vi "电机数据.vi"() -> ()   [LabVIEW 2017]
uses:
  LVMQTT/Controls/Connect_Flags.ctl
  LVMQTT/Controls/QoS.ctl
  <vilib>/Platform/TimedLoop/XDataNode/timing_clust.ctl
  <vilib>/Platform/TimedLoop/XDataNode/nitl_modes.ctl
  <vilib>/Platform/TimedLoop/XDataNode/wakeup.ctl
  <vilib>/Platform/TimedLoop/XDataNode/XDataNode.xnode
  LVMQTT/MQTT_Functions.lvlib
  <vilib>/Platform/TimedLoop/XDataNode/XDNodeRunTimeDep.lvlib
panel:
  out "波形":cluster{"扭矩":dbl, "扭矩":dbl, "扭矩":dbl}(graph)
  out "功率":dbl format="%#_10f"
  out "速度":dbl format="%#_10f"
  out "扭矩":dbl format="%#_10f"
  out "字符串":string
  in  "MQTT Broker":cluster{"address (IP)":string, "port":u16}={"address (IP)"="169.254.84.131", "port"=1883}
  out "period":u32
  out "period 2":u32
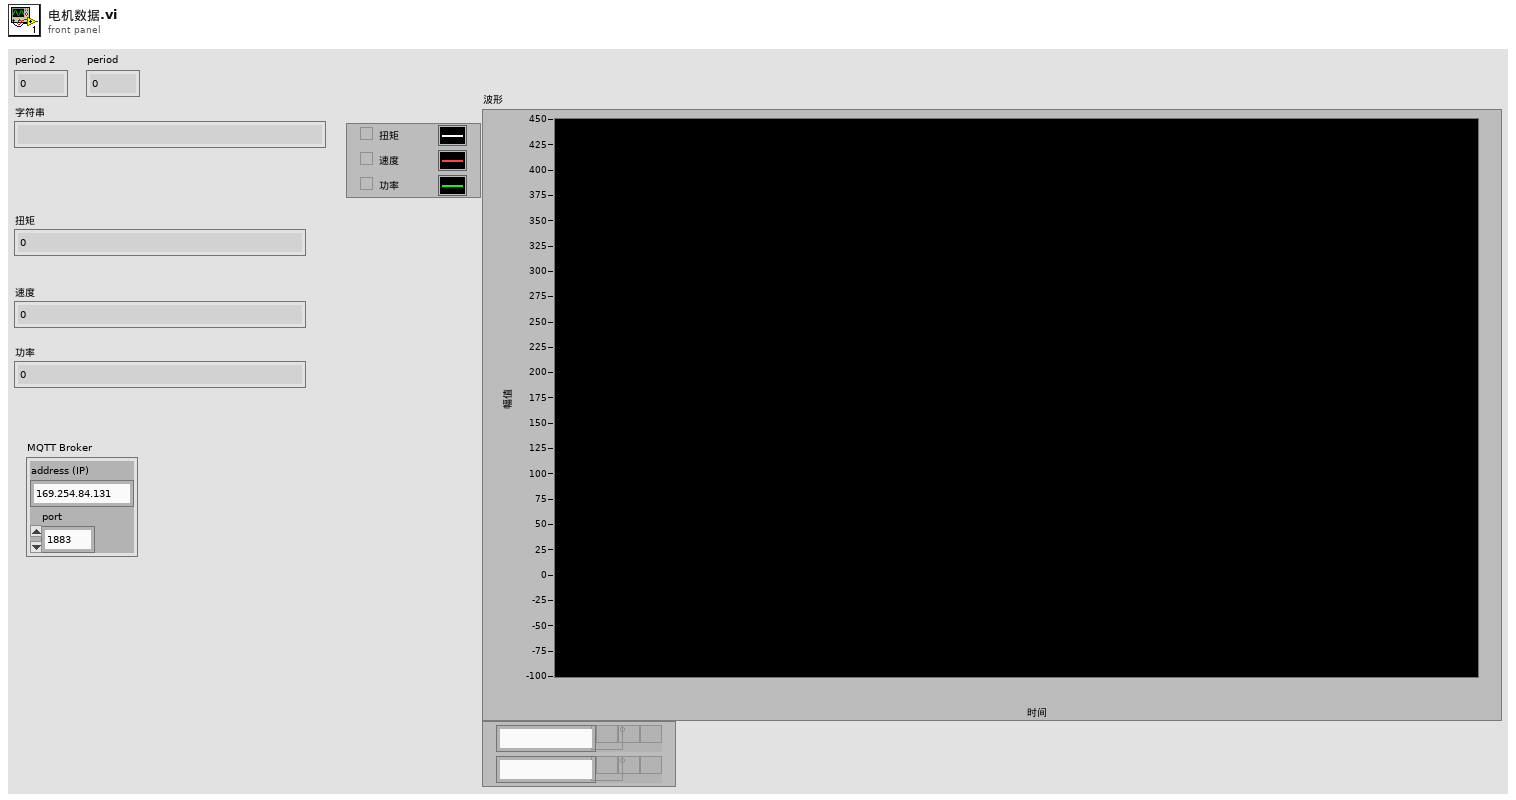
[diagram p1: front panel]
types:
  T1 = typedef "MQTT_Functions.lvlib/QoS.ctl" = enum8{"At most once", "At least once", "Exactly once", "Reserved"}
  T2 = typedef "MQTT_Functions.lvlib/Connect_Flags.ctl" = cluster{"user name":bool, "password":bool, "will retain":bool, "will flag":bool, "clean session":bool, "reserved":bool, "will QoS":T1}
  T3 = typedef "XDNodeRunTimeDep.lvlib/timing_clust.ctl" = cluster{"Expected End [f-1]":u64, "Actual End [f-1]":u64, "Finished Late? [f-1]":bool, "Expected End [i-1]":u64, "Actual End [i-1]":u64, "Finished Late? [i-1]":bool, "Expected Start [i]":u64, "Actual Start [i]":u64, "Expected Start [f]":u64, "Actual Start [f]":u64, "Source Name":string, "Structure Name":string, "Period":i64, "Deadline":i64, "Offset":i64, "Start":i64, "Priority":i32, "Timeout":i32, "Mode":T4, "Wakeup Reason":T5, "Error":errorcluster, "Source Type":string, "Secondary Source Type":string, "Global End Time":u64, "Global Start Time":u64, "Frame Duration":u64, "Iteration Duration":u64, "Assigned CPU":i32, "I/O Scan Engine Mode":u32}
  T4 = typedef "XDNodeRunTimeDep.lvlib/nitl_modes.ctl" = enum32{"No Change", "Process missed periods, maintain original phase", "Discard missed periods, maintain original phase", "Process missed periods, ignore original phase", "Discard missed periods, ignore original phase"}
  T5 = typedef "XDNodeRunTimeDep.lvlib/wakeup.ctl" = enum32{"Normal", "Aborted", "Asynchronous wakeup", "Timing source error", "Timed loop error", "Timeout"}
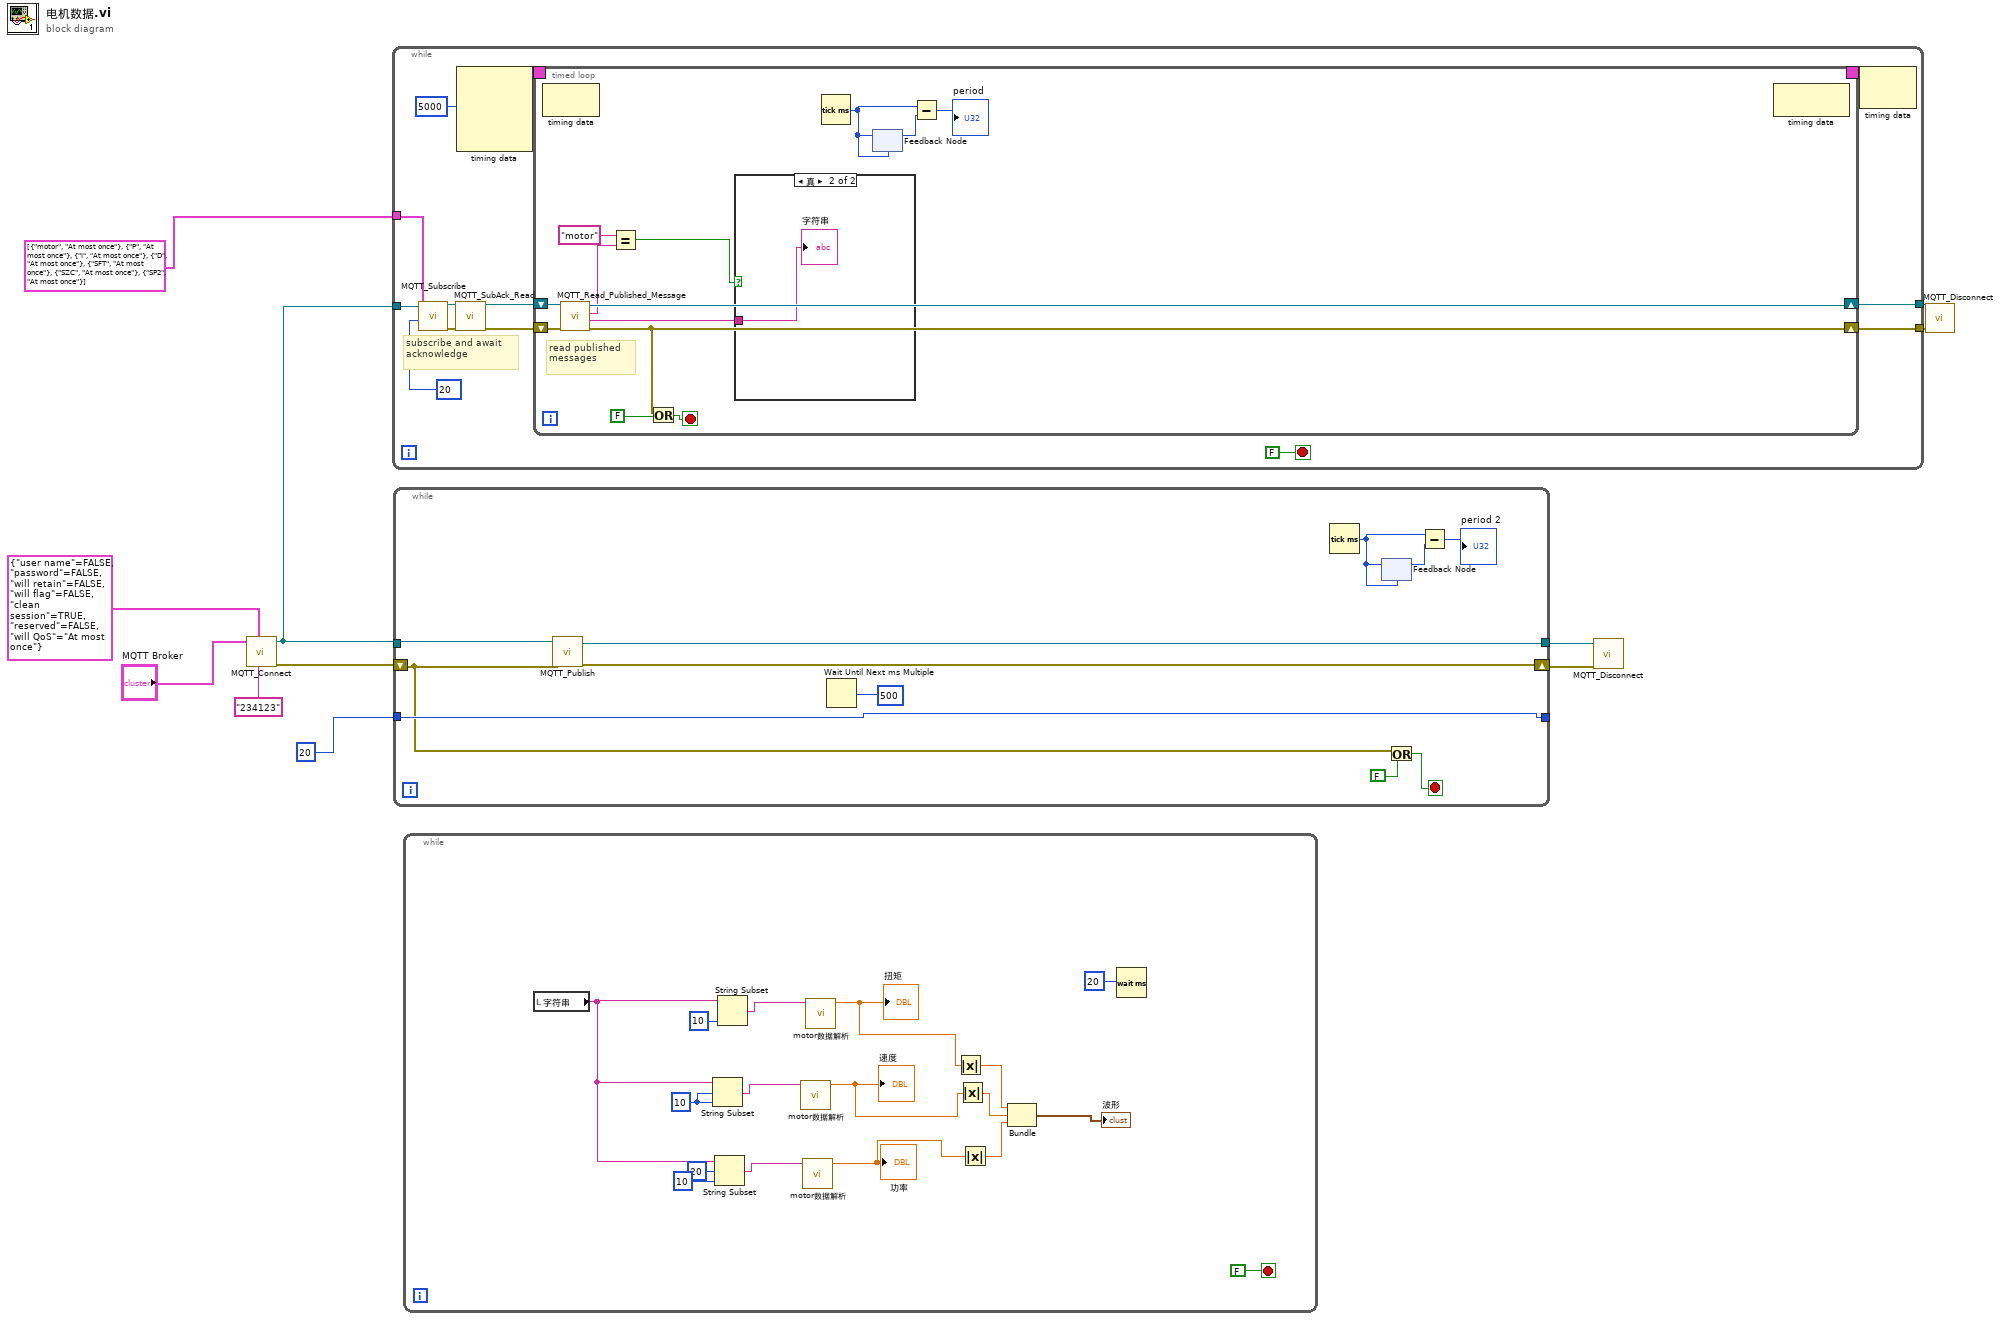
[diagram p0: block diagram]
diagram:
  n1 = call "MQTT_Connect.vi"("Client ID"="234123", "Connect Flags"=T2 {"user name"=FALSE, "password"=FALSE, "will retain"=FALSE, "will flag"=FALSE, "clean session"=TRUE, "reserved"=FALSE, "will QoS"=enum."At most once"}, "MQTT Broker"="MQTT Broker") -> ("error out"=w7:errorcluster, "connection ID out"=w6:refnum<k5>)  [unwired: 6 in, 1 out]
  n2 = while {
    tunnel: w6 -> [w19]
    tunnel: [w18] -> w3
    tunnel: [w17] -> w2
    tunnel: cluster{"Topic":string, "QoS":T1}[] [{"Topic"="motor", "QoS"=enum."At most once"}, {"Topic"="P", "QoS"=enum."At most once"}, {"Topic"="I", "QoS"=enum."At most once"}, {"Topic"="D", "QoS"=enum."At most once"}, {"Topic"="SFT", "QoS"=enum."At most once"}, {"Topic"="SZC", "QoS"=enum."At most once"}, {"Topic"="SP2", "QoS"=enum."At most once"}] ("Subscription Info Array") -> [w16]
    stop <- FALSE stop-if-true
    # "subscribe and await\nacknowledge"
    n3 = call "MQTT_Subscribe.vi"("Message ID"=u16 20, "Subscription Info Array"=w16, "connection ID"=w19) -> ("error out"=w22:errorcluster, "connection ID out"=w23:refnum<k5>)  [unwired: 7 in]
    n4 = call "MQTT_SubAck_Read.vi"("error in (no error)"=w22, "connection ID"=w23) -> ("error out"=w21:errorcluster, "connection ID out"=w20:refnum<k5>)  [unwired: 7 in, 1 out]
    n5 = node-c288(i64 5000 ("周期")) -> (w14:T3)  [unwired: 3 in]
    n6 = timed-loop {
      shift-right: [w29] -> w17
      shift-left: w21 -> [w37]
      shift-right: [w30] -> w18
      shift-left: w20 -> [w36]
      timing: w14 -> [_]
      timing-out: [_] -> w13
      stop <- w35 stop-if-true
      # "read published\nmessages"
      n7 = node-c288() -> ()  [unwired: 1 in, 1 out]
      n8 = call "MQTT_Read_Published_Message.vi"("error in (no error)"=w37, "connection ID"=w36) -> ("error out"=w29:errorcluster, "Message"=w28:string, "Topic Name"=w27:string, "connection ID out"=w30:refnum<k5>)  [unwired: 4 in, 2 out]
      n9 = Equal?(x="motor", y=w27) -> (x = y?=w25:bool)
      n10 = Or(x=w29, y=FALSE) -> (x .or. y?=w35:bool)
      n11 = case shown="真" w25 {
        tunnel: w28 -> [_ w38]
        frame False {
        }
        frame True {
          "字符串" <- w38
        }
      }
      n12 = Tick Count (ms)() -> (millisecond timer value=w33:u32)
      n13 = feedback #1(w33) -> (w31:u32)
      n14 = feedback-in #1(w33) -> ()
      n15 = Subtract(x=w33, y=w31) -> (x-y=→"period":u32)
      n16 = node-c288() -> ()  [unwired: 1 in, 1 out]
    }
    n17 = node-c288(w13) -> ()  [unwired: 1 out]
  }
  n18 = while {
    tunnel: [w45] -> w10
    tunnel: u16 20 ("Message ID") -> [w54]
    tunnel: [w54] -> _
    shift-right: [w46] -> w11
    shift-left: w7 -> [w47]
    tunnel: w6 -> [w48]
    stop <- w53 stop-if-true
    n19 = call "MQTT_Publish.vi"("error in (no error)"=w47, "connection ID"=w48) -> ("error out"=w46:errorcluster, "connection ID out"=w45:refnum<k5>)  [unwired: 8 in]
    n20 = Wait Until Next ms Multiple(millisecond multiple=u32 500) -> ()  [unwired: 1 out]
    n21 = Tick Count (ms)() -> (millisecond timer value=w51:u32)
    n22 = feedback #2(w51) -> (w49:u32)
    n23 = feedback-in #2(w51) -> ()
    n24 = Or(x=w47, y=FALSE) -> (x .or. y?=w53:bool)
    n25 = Subtract(x=w51, y=w49) -> (x-y=→"period 2":u32)
  }
  n26 = while {
    stop <- FALSE stop-if-true
    w67 = 10 ("长度（剩余）")
    n27 = local read "字符串"() -> (w64:string)
    n28 = String Subset(string=w64, offset (0)=w67, length (rest)=w67) -> (substring=w68:string)
    n29 = String Subset(string=w64, offset (0)=20 ("偏移量(0)"), length (rest)=10 ("长度（剩余）")) -> (substring=w65:string)
    n30 = String Subset(string=w64, length (rest)=10 ("长度（剩余）")) -> (substring=w69:string)  [unwired: 1 in]
    n31 = call "motor数据解析.vi"("字符串"=w68) -> ("扭矩"=w58:dbl)  [unwired: 10 in]
    "速度" <- w58
    n32 = call "motor数据解析.vi"("字符串"=w65) -> ("扭矩"=w56:dbl)  [unwired: 10 in]
    "功率" <- w56
    n33 = call "motor数据解析.vi"("字符串"=w69) -> ("扭矩"=w61:dbl)  [unwired: 10 in]
    "扭矩" <- w61
    n34 = Absolute Value(x=w61) -> (abs(x)=w60:dbl)
    n35 = Absolute Value(x=w58) -> (abs(x)=w59:dbl)
    n36 = Absolute Value(x=w56) -> (abs(x)=w57:dbl)
    n37 = Bundle(w60, w59, w57) -> (→"波形":cluster{dbl, dbl, dbl})  [unwired: 1 in]
    n38 = Wait (ms)(milliseconds to wait=u32 20 ("等待时间（毫秒）")) -> ()  [unwired: 1 out]
  }
  n39 = call "MQTT_Disconnect.vi"("error in (no error)"=w11, "connection ID"=w10) -> ()  [unwired: 9 in, 1 out]
  n40 = call "MQTT_Disconnect.vi"("error in (no error)"=w2, "connection ID"=w3) -> ()  [unwired: 9 in, 1 out]
